vi "Input Output AC Signal Test.vi"() -> ()   [LabVIEW 2012]
uses:
  <vilib>/rvi/FXPMathLib/FxpSinAndCos/subVIs/nifxpmath_SinAndCos_SimConfig.ctl
  <vilib>/rvi/FXPMathLib/FxpSinAndCos/simVIs/DllFxpSinAndCosTemp_sub.vi
  <vilib>/rvi/eio/common/nirviEmuTemplateMethod_errors.vi
  <vilib>/rvi/FXPMathLib/FxpSinAndCos/XNode/nifxpmath_SinAndCos.xnode
  <vilib>/eio/EIONode/EIONode.xnode
panel:
  out "Numeric 2":i16
  out "Numeric":sgl
  out "Input Signal":fxp<+/-,26,16>
  in  "Start":bool
  out "Output Signal":fxp<+/-,26,16>
  in  "Phase Shift":fxp<+/-,19,16>
  in  "Frequency":i16
  in  "Voltage":fxp<+/-,25,16>
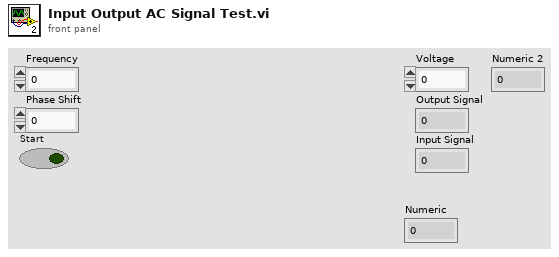
[diagram p1: front panel]
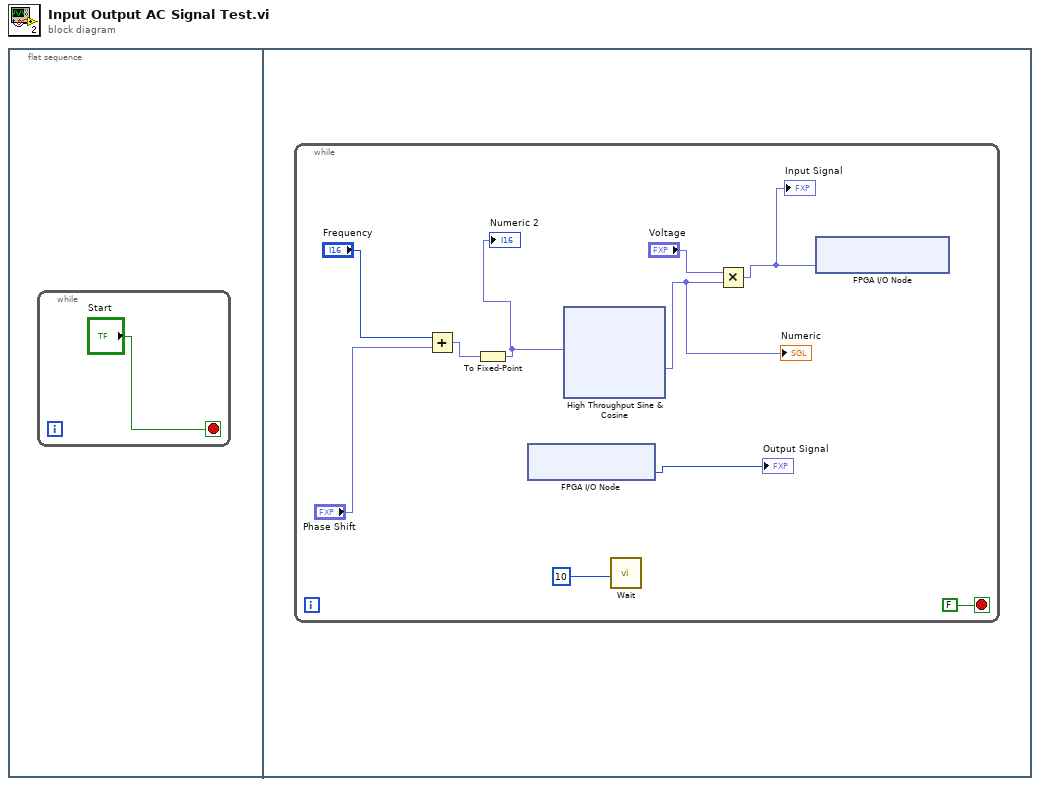
[diagram p0: block diagram]
diagram:
  n1 = flat-sequence {
    frame #0 {
      n2 = while {
        stop <- "Start" stop-if-true
      }
    }
    frame #1 {
      n3 = while {
        stop <- FALSE stop-if-true
        n4 = Add(x="Frequency", y="Phase Shift") -> (x+y=w9:fxp<+/-,20,17>)
        n5 = To Fixed-Point(number=w9) -> (fixed-point=w2:fxp<+/-,20,17>)  [unwired: 1 in]
        "Numeric 2" <- w2
        n6 = xnode "FPGA I/O Node"() -> ("Connector0/AI4"=→"Output Signal":i16)  [unwired: 1 in, 1 out]
        n7 = xnode "High Throughput Sine & Cosine"("x (pi)"=w2) -> ("sin(x)"=w3:fxp<+/-,16,2>)  [unwired: 1 out]
        "Numeric" <- w3
        n8 = call "Wait"("Count(mSec)"=i16 10) -> ()  [unwired: 1 out]
        n9 = Multiply(x="Voltage", y=w3) -> (x*y=w6:fxp<+/-,41,18>)
        "Input Signal" <- w6
        n10 = xnode "FPGA I/O Node"("Connector0/AO4"=w6) -> ()  [unwired: 1 in, 1 out]
      }
    }
  }
